vi "onHttpPost (File).vi"(6 "timeout":i32=10000, 7 "output file":path, 8 "error in":errorcluster, 9 "file":path, 10 "url":string, 11 "http-method in":refnum<class "basic-http-client.lvclass">) -> (0 "error out":errorcluster, 1 "body":string, 2 "headers":string, 3 "http-method out":refnum<class "basic-http-client.lvclass">)   [LabVIEW 2020, in "REST Client.lvlib" / "basic-http-client.lvclass"]
uses:
  basic-http-client.lvclass
  basic-http-client.lvclass/basic-http-client.ctl
  <vilib>/httpClient/LabVIEWHTTPClient.lvlib
  <vilib>/httpClient/POSTFile.vi
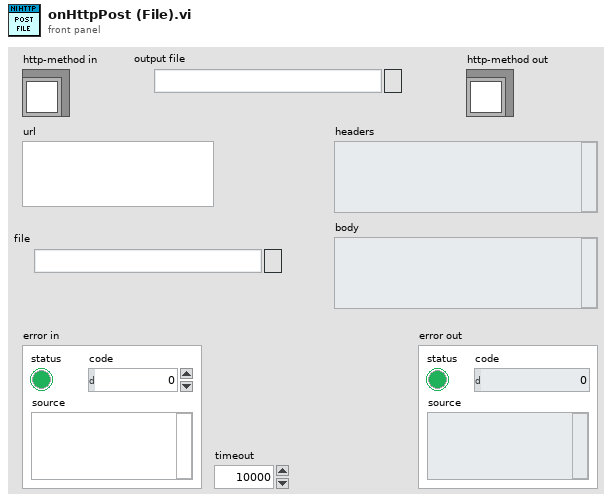
[diagram p1: front panel]
types:
  T1 = typedef "LabVIEWHTTPClient.lvlib/ClientHandle.ctl" = refnum<k1>
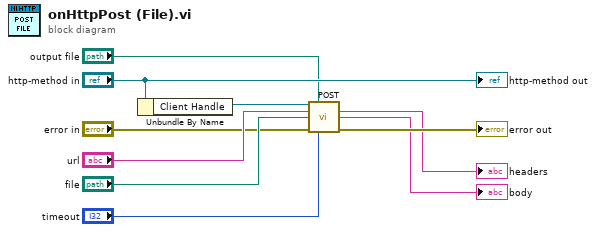
[diagram p0: block diagram]
diagram:
  n1 = Unbundle By Name("http-method in") -> ("Client Handle"=w9:T1)
  n2 = call-poly <vilib>:"POST.vi"("client handle"=w9, "output file"="output file", "url"="url", "file"="file", "error in (no error)"="error in", "timeout (10000)"="timeout") -> ("headers"=→"headers":string, "body"=→"body":string, "error out"=→"error out":errorcluster)  [unwired: 6 in, 1 out]
  "http-method out" <- "http-method in"
